vi "shared memory read.vi"(8 "error in":errorcluster, 9 "File Array":dbl[](array[numeric]), 10 "Data Array":dbl[](array[numeric]), 11 "refnum in":refnum<file>) -> (0 "error out":errorcluster, 1 "File Array out":dbl[](array[numeric]), 2 "Data Array out":dbl[](array[numeric]), 3 "refnum out":refnum<file>, 4 "data valid?":bool)   [LabVIEW 2013, in "current tag file io module runtime.lvclass"]
uses:
  current tag file io module runtime.lvclass
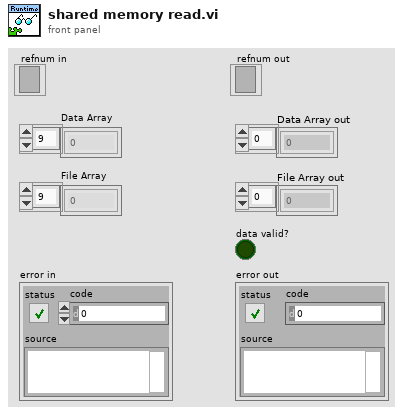
[diagram p1: front panel]
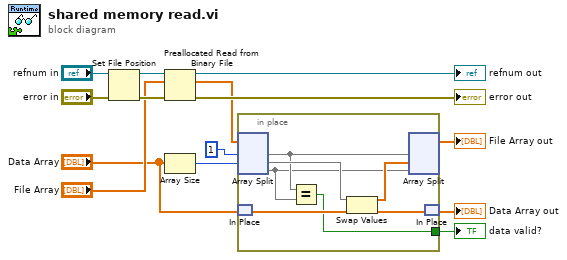
[diagram p0: block diagram]
diagram:
  n1 = Set File Position(refnum="refnum in", error in="error in") -> (refnum out=w11:refnum<file>, error out=w10:errorcluster)  [unwired: 2 in]
  n2 = Preallocated Read from Binary File(4:w10, 6:"File Array", 7:w11) -> (0:→"error out":errorcluster, 2:w7:dbl[], 3:→"refnum out":refnum<file>)  [unwired: 1 in, 1 out]
  n3 = Array Size(array="Data Array") -> (size(s)=w4:i32)
  n4 = in-place {
    in-place-border: [w15] -> w1
    n5 = in-place-split #1(w7, 1, w4) -> (w17:dbl[], w21:dbl[], w16:dbl[])
    n6 = in-place-match #2("Data Array") -> (w20:dbl[])
    n7 = Equal?(x=w17, y=w16) -> (x = y?=w15:bool)
    n8 = Swap Values(12:w21, 14:w20) -> (1:w18:dbl[], 3:w19:dbl[])  [unwired: 1 in]
    n9 = in-place-split #1(w17, w18, w16) -> (→"File Array out":dbl[])  [unwired: 2 out]
    n10 = in-place-match #2(w19) -> (→"Data Array out":dbl[])
  }
  "data valid?" <- w1
